vi "Main.vi"(7 "sweep rate, /min":dbl=0.2, 8 "sweep to:":dbl=-0.5, 9 "sweep":T3(radio)=enum."time_sweep") -> ()   [LabVIEW 2017] (continued)
                      n1646 = Number To Decimal String(number=w2143) -> (decimal integer string=w2142:string)  [unwired: 1 in]
                      n1647 = GPIB Write(0:w2142, 1:":SENSe:DATA:FRES?") -> (6:w2147:errorcluster)  [unwired: 3 in, 1 out]
                      n1648 = GPIB Read(0:w2142, 1:200, 3:w2147) -> (5:w2141:string)  [unwired: 2 in, 2 out]
                      n1649 = Fract/Exp String To Number(string=w2141) -> (number=w2145:dbl)  [unwired: 3 in, 1 out]
                      n1650 = Build Array (concatenate)(w2149, w2145) -> (w2148:dbl[])
                    }
                  }
                  n1651 = property on="data" class="Arr (strict)"("Value"=w2139) -> ()  [unwired: 2 in, 2 out]
                }
                frame #17 {
                  # "check if 2nd channel \non Keithley 2182A 2\nis to be measured"
                  n1652 = property on="data" class="Arr (strict)"() -> ("Value"=w2151:dbl[])  [unwired: 2 in, 2 out]
                  n1653 = local read "2182A 2 ch2"() -> (w2150:bool)
                  n1654 = case shown="True" w2150 {
                    tunnel: w2151 -> [w2153 w2166]
                    tunnel: [w2153 w2165] -> w2152
                    frame False {
                      # "we are not measuring 2182A 2 channel 2 (2182A_2_ch2)"
                    }
                    frame True {
                      # "switching to channel 2 and then\nback to channel 1"
                      # "we are  measuring 2182A 2 channel 2 (2182A_2_ch2)"
                      n1655 = local read "2182A 2 addr"() -> (w2160:u8)
                      n1656 = Number To Decimal String(number=w2160) -> (decimal integer string=w2155:string)  [unwired: 1 in]
                      n1657 = GPIB Write(0:w2155, 1:":SENSe:CHAN 2") -> (6:w2157:errorcluster)  [unwired: 3 in, 1 out]
                      n1658 = GPIB Write(0:w2155, 1:":SENSe:DATA:FRES?", 3:w2157) -> (6:w2164:errorcluster)  [unwired: 2 in, 1 out]
                      n1659 = GPIB Read(0:w2155, 1:200, 3:w2164) -> (5:w2159:string, 7:w2156:errorcluster)  [unwired: 2 in, 1 out]
                      n1660 = GPIB Write(0:w2155, 1:":SENSe:CHAN 1", 3:w2156) -> ()  [unwired: 2 in, 2 out]
                      n1661 = Fract/Exp String To Number(string=w2159) -> (number=w2162:dbl)  [unwired: 3 in, 1 out]
                      n1662 = Build Array (concatenate)(w2166, w2162) -> (w2165:dbl[])
                    }
                  }
                  n1663 = property on="data" class="Arr (strict)"("Value"=w2152) -> ()  [unwired: 2 in, 2 out]
                }
                frame #18 {
                  # "check if 1st channel \non Keithley 2182A 3\nis to be measured"
                  n1664 = property on="data" class="Arr (strict)"() -> ("Value"=w2168:dbl[])  [unwired: 2 in, 2 out]
                  n1665 = local read "2182A 3 ch1"() -> (w2167:bool)
                  n1666 = case shown="True" w2167 {
                    tunnel: w2168 -> [w2170 w2179]
                    tunnel: [w2170 w2178] -> w2169
                    frame False {
                      # "we are not measuring 2182A 3 channel 1 (2182A_3_ch1)"
                    }
                    frame True {
                      # "we are  measuring 2182A 3 channel 1 (2182A_3_ch1)"
                      n1667 = local read "2182A 3 addr"() -> (w2173:u8)
                      n1668 = Number To Decimal String(number=w2173) -> (decimal integer string=w2172:string)  [unwired: 1 in]
                      n1669 = GPIB Write(0:w2172, 1:":SENSe:DATA:FRES?") -> (6:w2177:errorcluster)  [unwired: 3 in, 1 out]
                      n1670 = GPIB Read(0:w2172, 1:200, 3:w2177) -> (5:w2171:string)  [unwired: 2 in, 2 out]
                      n1671 = Fract/Exp String To Number(string=w2171) -> (number=w2175:dbl)  [unwired: 3 in, 1 out]
                      n1672 = Build Array (concatenate)(w2179, w2175) -> (w2178:dbl[])
                    }
                  }
                  n1673 = property on="data" class="Arr (strict)"("Value"=w2169) -> ()  [unwired: 2 in, 2 out]
                }
                frame #19 {
                  # "check if 2nd channel \non Keithley 2182A 3\nis to be measured"
                  n1674 = property on="data" class="Arr (strict)"() -> ("Value"=w2181:dbl[])  [unwired: 2 in, 2 out]
                  n1675 = local read "2182A 3 ch2"() -> (w2180:bool)
                  n1676 = case shown="True" w2180 {
                    tunnel: w2181 -> [w2183 w2196]
                    tunnel: [w2183 w2195] -> w2182
                    frame False {
                      # "we are not measuring 2182A 3 channel 2 (2182A_3_ch2)"
                    }
                    frame True {
                      # "switching to channel 2 and then\nback to channel 1"
                      # "we are  measuring 2182A 3 channel 2 (2182A_3_ch2)"
                      n1677 = local read "2182A 3 addr"() -> (w2190:u8)
                      n1678 = Number To Decimal String(number=w2190) -> (decimal integer string=w2185:string)  [unwired: 1 in]
                      n1679 = GPIB Write(0:w2185, 1:":SENSe:CHAN 2") -> (6:w2187:errorcluster)  [unwired: 3 in, 1 out]
                      n1680 = GPIB Write(0:w2185, 1:":SENSe:DATA:FRES?", 3:w2187) -> (6:w2194:errorcluster)  [unwired: 2 in, 1 out]
                      n1681 = GPIB Read(0:w2185, 1:200, 3:w2194) -> (5:w2189:string, 7:w2186:errorcluster)  [unwired: 2 in, 1 out]
                      n1682 = GPIB Write(0:w2185, 1:":SENSe:CHAN 1", 3:w2186) -> ()  [unwired: 2 in, 2 out]
                      n1683 = Fract/Exp String To Number(string=w2189) -> (number=w2192:dbl)  [unwired: 3 in, 1 out]
                      n1684 = Build Array (concatenate)(w2196, w2192) -> (w2195:dbl[])
                    }
                  }
                  n1685 = property on="data" class="Arr (strict)"("Value"=w2182) -> ()  [unwired: 2 in, 2 out]
                }
                frame #20 {
                  # "check if 1st channel \non Keithley 2182A 4\nis to be measured"
                  n1686 = property on="data" class="Arr (strict)"() -> ("Value"=w2198:dbl[])  [unwired: 2 in, 2 out]
                  n1687 = local read "2182A 4 ch1"() -> (w2197:bool)
                  n1688 = case shown="True" w2197 {
                    tunnel: w2198 -> [w2200 w2209]
                    tunnel: [w2200 w2208] -> w2199
                    frame False {
                      # "we are not measuring 2182A 4 channel 1 (2182A_4_ch1)"
                    }
                    frame True {
                      # "we are  measuring 2182A 4 channel 1 (2182A_4_ch1)"
                      n1689 = local read "2182A 4 addr"() -> (w2203:u8)
                      n1690 = Number To Decimal String(number=w2203) -> (decimal integer string=w2202:string)  [unwired: 1 in]
                      n1691 = GPIB Write(0:w2202, 1:":SENSe:DATA:FRES?") -> (6:w2207:errorcluster)  [unwired: 3 in, 1 out]
                      n1692 = GPIB Read(0:w2202, 1:200, 3:w2207) -> (5:w2201:string)  [unwired: 2 in, 2 out]
                      n1693 = Fract/Exp String To Number(string=w2201) -> (number=w2205:dbl)  [unwired: 3 in, 1 out]
                      n1694 = Build Array (concatenate)(w2209, w2205) -> (w2208:dbl[])
                    }
                  }
                  n1695 = property on="data" class="Arr (strict)"("Value"=w2199) -> ()  [unwired: 2 in, 2 out]
                }
                frame #21 {
                  # "check if 2nd channel \non Keithley 2182A 4\nis to be measured"
                  n1696 = property on="data" class="Arr (strict)"() -> ("Value"=w2211:dbl[])  [unwired: 2 in, 2 out]
                  n1697 = local read "2182A 4 ch2"() -> (w2210:bool)
                  n1698 = case shown="True" w2210 {
                    tunnel: w2211 -> [w2213 w2226]
                    tunnel: [w2213 w2225] -> w2212
                    frame False {
                      # "we are not measuring 2182A 4 channel 2 (2182A_4_ch2)"
                    }
                    frame True {
                      # "switching to channel 2 and then\nback to channel 1"
                      # "we are  measuring 2182A 4 channel 2 (2182A_4_ch2)"
                      n1699 = local read "2182A 4 addr"() -> (w2220:u8)
                      n1700 = Number To Decimal String(number=w2220) -> (decimal integer string=w2215:string)  [unwired: 1 in]
                      n1701 = GPIB Write(0:w2215, 1:":SENSe:CHAN 2") -> (6:w2217:errorcluster)  [unwired: 3 in, 1 out]
                      n1702 = GPIB Write(0:w2215, 1:":SENSe:DATA:FRES?", 3:w2217) -> (6:w2224:errorcluster)  [unwired: 2 in, 1 out]
                      n1703 = GPIB Read(0:w2215, 1:200, 3:w2224) -> (5:w2219:string, 7:w2216:errorcluster)  [unwired: 2 in, 1 out]
                      n1704 = GPIB Write(0:w2215, 1:":SENSe:CHAN 1", 3:w2216) -> ()  [unwired: 2 in, 2 out]
                      n1705 = Fract/Exp String To Number(string=w2219) -> (number=w2222:dbl)  [unwired: 3 in, 1 out]
                      n1706 = Build Array (concatenate)(w2226, w2222) -> (w2225:dbl[])
                    }
                  }
                  n1707 = property on="data" class="Arr (strict)"("Value"=w2212) -> ()  [unwired: 2 in, 2 out]
                }
                frame #22 {
                  # "check if voltage on\nKeithley 2636A smua\nis to be measured"
                  n1708 = local read "2636A smua meas v"() -> (w2227:bool)
                  n1709 = property on="data" class="Arr (strict)"() -> ("Value"=w2228:dbl[])  [unwired: 2 in, 2 out]
                  n1710 = case shown="True" w2227 {
                    tunnel: w2228 -> [w2230 w2236]
                    tunnel: [w2230 w2235] -> w2229
                    frame False {
                      # "we are not measuring voltage on 2636A smua (2636A_smua_v)"
                    }
                    frame True {
                      # "we are  measuring voltage on 2636A smua (2636A_smua_v)"
                      n1711 = local read "2336A addr"() -> (w2231:refnum<visa-resource-name>)
                      n1712 = call "SinglePointMeasurement.vi"("Measure"=Measure."Voltage", "Channel"=Channel."a", "VISA resource name 2"=w2231) -> ("Measuremet"=w2233:dbl)  [unwired: 3 in, 4 out]
                      n1713 = Build Array (concatenate)(w2236, w2233) -> (w2235:dbl[])
                    }
                  }
                  n1714 = property on="data" class="Arr (strict)"("Value"=w2229) -> ()  [unwired: 2 in, 2 out]
                }
                frame #23 {
                  # "check if current on\nKeithley 2636A smua\nis to be measured"
                  n1715 = local read "2636A smua meas i"() -> (w2237:bool)
                  n1716 = property on="data" class="Arr (strict)"() -> ("Value"=w2238:dbl[])  [unwired: 2 in, 2 out]
                  n1717 = case shown="True" w2237 {
                    tunnel: w2238 -> [w2240 w2243]
                    tunnel: [w2240 w2242] -> w2239
                    frame False {
                      # "we are not measuring current on 2636A smua (2636A_smua_i)"
                    }
                    frame True {
                      # "we are  measuring current on 2636A smua (2636A_smua_i)"
                      n1718 = stacked-sequence {
                        tunnel: [_ w2252] -> w2241
                        frame #0 {
                          n1719 = local read "auto\nrange A"() -> (w2247:bool)
                          n1720 = local read "2336A addr"() -> (w2250:refnum<visa-resource-name>)
                          n1721 = Select(t="smua.AUTORANGE_ON", s=w2247, f="smua.AUTORANGE_OFF") -> (s? t:f=w2245:string)
                          n1722 = Concatenate Strings("smua.measure.autorangei = ", w2245) -> (w2244:string)
                          n1723 = VISA Write(VISA resource name=w2250, write buffer=w2244) -> ()  [unwired: 1 in, 3 out]
                        }
                        frame #1 {
                          n1724 = local read "2336A addr"() -> (w2254:refnum<visa-resource-name>)
                          n1725 = call "SinglePointMeasurement.vi"("Measure"=Measure."Current", "Channel"=Channel."a", "VISA resource name 2"=w2254) -> ("Measuremet"=w2252:dbl)  [unwired: 3 in, 4 out]
                        }
                      }
                      n1726 = Build Array (concatenate)(w2243, w2241) -> (w2242:dbl[])
                    }
                  }
                  n1727 = property on="data" class="Arr (strict)"("Value"=w2239) -> ()  [unwired: 2 in, 2 out]
                }
                frame #24 {
                  # "check if voltage on\nKeithley 2636A smub\nis to be measured"
                  n1728 = local read "2636A smub meas v"() -> (w2255:bool)
                  n1729 = property on="data" class="Arr (strict)"() -> ("Value"=w2256:dbl[])  [unwired: 2 in, 2 out]
                  n1730 = case shown="True" w2255 {
                    tunnel: w2256 -> [w2258 w2264]
                    tunnel: [w2258 w2263] -> w2257
                    frame False {
                      # "we are not measuring voltage on 2636A smub (2636A_smub_v)"
                    }
                    frame True {
                      # "we are  measuring voltage on 2636A smub (2636A_smub_v)"
                      n1731 = local read "2336A addr"() -> (w2262:refnum<visa-resource-name>)
                      n1732 = call "SinglePointMeasurement.vi"("Measure"=Measure."Voltage", "Channel"=Channel."b", "VISA resource name 2"=w2262) -> ("Measuremet"=w2260:dbl)  [unwired: 3 in, 4 out]
                      n1733 = Build Array (concatenate)(w2264, w2260) -> (w2263:dbl[])
                    }
                  }
                  n1734 = property on="data" class="Arr (strict)"("Value"=w2257) -> ()  [unwired: 2 in, 2 out]
                }
                frame #25 {
                  # "check if current on\nKeithley 2636A smub\nis to be measured"
                  n1735 = local read "2636A smub meas i"() -> (w2265:bool)
                  n1736 = property on="data" class="Arr (strict)"() -> ("Value"=w2266:dbl[])  [unwired: 2 in, 2 out]
                  n1737 = case shown="True" w2265 {
                    tunnel: w2266 -> [w2268 w2271]
                    tunnel: [w2268 w2270] -> w2267
                    frame False {
                      # "we are not measuring current on 2636A smub (2636A_smub_i)"
                    }
                    frame True {
                      # "we are  measuring current on 2636A smub (2636A_smub_i)"
                      n1738 = stacked-sequence {
                        tunnel: [_ w2280] -> w2269
                        frame #0 {
                          n1739 = local read "auto\nrange B"() -> (w2275:bool)
                          n1740 = local read "2336A addr"() -> (w2278:refnum<visa-resource-name>)
                          n1741 = Select(t="smub.AUTORANGE_ON", s=w2275, f="smub.AUTORANGE_OFF") -> (s? t:f=w2273:string)
                          n1742 = Concatenate Strings("smub.measure.autorangei = ", w2273) -> (w2272:string)
                          n1743 = VISA Write(VISA resource name=w2278, write buffer=w2272) -> ()  [unwired: 1 in, 3 out]
                        }
                        frame #1 {
                          n1744 = local read "2336A addr"() -> (w2282:refnum<visa-resource-name>)
                          n1745 = call "SinglePointMeasurement.vi"("Measure"=Measure."Current", "Channel"=Channel."b", "VISA resource name 2"=w2282) -> ("Measuremet"=w2280:dbl)  [unwired: 3 in, 4 out]
                        }
                      }
                      n1746 = Build Array (concatenate)(w2271, w2269) -> (w2270:dbl[])
                    }
                  }
                  n1747 = property on="data" class="Arr (strict)"("Value"=w2267) -> ()  [unwired: 2 in, 2 out]
                }
                frame #26 {
                  # "check if time\nis to be measured"
                  n1748 = property on="data" class="Arr (strict)"() -> ("Value"=w2285:dbl[])  [unwired: 2 in, 2 out]
                  n1749 = local read "measure time"() -> (w2284:bool)
                  n1750 = case shown="True" w2284 {
                    tunnel: w2285 -> [w2287 w2293]
                    tunnel: [w2287 w2292] -> w2286
                    tunnel: w2283 -> [_ w2290]
                    frame False {
                      # "we are not measuring time"
                    }
                    frame True {
                      # "seconds from the beginning of month"
                      # "we are  measuring time"
                      n1751 = call "timeInSeconds.vi"() -> ("Numeric"=w2291:dbl, "current time"=w2288:timestamp)  [unwired: 2 in]
                      n1752 = property on="current time" class="AbsTime (strict)"("Value"=w2288) -> ()  [unwired: 2 in, 2 out]
                      n1753 = Subtract(x=w2291, y=w2290) -> (x-y=w2289:dbl)
                      n1754 = Build Array (concatenate)(w2293, w2289) -> (w2292:dbl[])
                    }
                  }
                  n1755 = property on="data" class="Arr (strict)"("Value"=w2286) -> ()  [unwired: 2 in, 2 out]
                }
                frame #27 {
                  n1756 = local read "iPS_MagnetField"() -> (w2294:bool)
                  n1757 = property on="data" class="Arr (strict)"() -> ("Value"=w2295:dbl[])  [unwired: 2 in, 2 out]
                  n1758 = case shown="True" w2294 {
                    tunnel: w2295 -> [w2297 w2306]
                    tunnel: [w2297 w2305] -> w2296
                    frame False {
                      # "we are not Measuring magnetic field on IPS120-0"
                    }
                    frame True {
                      w2301 = 1
                      # "Measure magnetic field on Teslatron_iPS_Field"
                      n1759 = local read "IPS120-0 addr_sweep"() -> (w2304:u8)
                      n1760 = Number To Decimal String(number=w2304) -> (decimal integer string=w2303:string)  [unwired: 1 in]
                      n1761 = GPIB Write(0:w2303, 1:"R 7", 2:w2301) -> ()  [unwired: 2 in, 2 out]
                      n1762 = GPIB Read(0:w2303, 1:200 ("byte count"), 2:w2301) -> (5:w2299:string)  [unwired: 2 in, 2 out]
                      n1763 = Fract/Exp String To Number(string=w2299, offset=w2301) -> (number=w2300:dbl)  [unwired: 2 in, 1 out]
                      n1764 = Build Array (concatenate)(w2306, w2300) -> (w2305:dbl[])
                    }
                  }
                  n1765 = property on="data" class="Arr (strict)"("Value"=w2296) -> ()  [unwired: 2 in, 2 out]
                }
                frame #28 {
                  # "check if current \non 2461 SouceMeter\nis to be measured"
                  n1766 = property on="data" class="Arr (strict)"() -> ("Value"=w2308:dbl[])  [unwired: 2 in, 2 out]
                  n1767 = property on="iTC_Sample_T" class="Bool (strict)"() -> ("Value"=w2307:bool)  [unwired: 2 in, 2 out]
                  n1768 = case shown="True" w2307 {
                    tunnel: w2308 -> [w2310 w2323]
                    tunnel: [w2310 w2322] -> w2309
                    frame False {
                      # "we are not measuring 2461, voltage (2461_meas_v)"
                    }
                    frame True {
                      w2316 = 1
                      # "temporarily ITC503S"
                      # "we are  measuring Sample_T"
                      n1769 = property on="iTC_503_addr_sweep" class="DigNum (strict)"() -> ("Value"=w2311:u8)  [unwired: 2 in, 2 out]
                      n1770 = Number To Decimal String(number=w2311) -> (decimal integer string=w2312:string)  [unwired: 1 in]
                      n1771 = GPIB Write(0:w2312, 1:"$C3", 2:1) -> (6:w2319:errorcluster)  [unwired: 2 in, 1 out]
                      n1772 = GPIB Write(0:w2312, 1:"R3", 2:w2316, 3:w2319) -> (6:w2321:errorcluster)  [unwired: 1 in, 1 out]
                      n1773 = GPIB Read(0:w2312, 1:200, 2:w2316, 3:w2321) -> (5:w2320:string)  [unwired: 1 in, 2 out]
                      n1774 = Fract/Exp String To Number(string=w2320, offset=w2316) -> (number=w2313:dbl)  [unwired: 2 in, 1 out]
                      n1775 = Build Array (concatenate)(w2323, w2313) -> (w2322:dbl[])
                    }
                  }
                  n1776 = property on="data" class="Arr (strict)"("Value"=w2309) -> ()  [unwired: 2 in, 2 out]
                }
                frame #29 {
                  # "check if current \non 2461 SouceMeter\nis to be measured"
                  n1777 = property on="CH_A" class="Bool (strict)"() -> ("Value"=w2324:bool)  [unwired: 2 in, 2 out]
                  n1778 = property on="data" class="Arr (strict)"() -> ("Value"=w2325:dbl[])  [unwired: 2 in, 2 out]
                  n1779 = case shown="True" w2324 {
                    tunnel: w2325 -> [w2327 w2340]
                    tunnel: [w2327 w2339] -> w2326
                    frame False {
                      # "we are not measuring 2461, voltage (2461_meas_v)"
                    }
                    frame True {
                      w2333 = 1
                      # "temporarily ITC503S"
                      # "we are  measuring iTC503_CHA"
                      n1780 = property on="iTC_503_addr_sweep" class="DigNum (strict)"() -> ("Value"=w2328:u8)  [unwired: 2 in, 2 out]
                      n1781 = Number To Decimal String(number=w2328) -> (decimal integer string=w2329:string)  [unwired: 1 in]
                      n1782 = GPIB Write(0:w2329, 1:"$C3", 2:1) -> (6:w2336:errorcluster)  [unwired: 2 in, 1 out]
                      n1783 = GPIB Write(0:w2329, 1:"R3", 2:w2333, 3:w2336) -> (6:w2338:errorcluster)  [unwired: 1 in, 1 out]
                      n1784 = GPIB Read(0:w2329, 1:200, 2:w2333, 3:w2338) -> (5:w2337:string)  [unwired: 1 in, 2 out]
                      n1785 = Fract/Exp String To Number(string=w2337, offset=w2333) -> (number=w2330:dbl)  [unwired: 2 in, 1 out]
                      n1786 = Build Array (concatenate)(w2340, w2330) -> (w2339:dbl[])
                    }
                  }
                  n1787 = property on="data" class="Arr (strict)"("Value"=w2326) -> ()  [unwired: 2 in, 2 out]
                }
                frame #30 {
                  # "check if current \non 2461 SouceMeter\nis to be measured"
                  n1788 = property on="CH_B" class="Bool (strict)"() -> ("Value"=w2341:bool)  [unwired: 2 in, 2 out]
                  n1789 = property on="data" class="Arr (strict)"() -> ("Value"=w2342:dbl[])  [unwired: 2 in, 2 out]
                  n1790 = case shown="True" w2341 {
                    tunnel: w2342 -> [w2344 w2357]
                    tunnel: [w2344 w2356] -> w2343
                    frame False {
                      # "we are not measuring 2461, voltage (2461_meas_v)"
                    }
                    frame True {
                      w2350 = 1
                      # "temporarily ITC503S"
                      # "we are  measuring iTC503_CHA"
                      n1791 = property on="iTC_503_addr_sweep" class="DigNum (strict)"() -> ("Value"=w2345:u8)  [unwired: 2 in, 2 out]
                      n1792 = Number To Decimal String(number=w2345) -> (decimal integer string=w2346:string)  [unwired: 1 in]
                      n1793 = GPIB Write(0:w2346, 1:"$C3", 2:1) -> (6:w2353:errorcluster)  [unwired: 2 in, 1 out]
                      n1794 = GPIB Write(0:w2346, 1:"R2", 2:w2350, 3:w2353) -> (6:w2355:errorcluster)  [unwired: 1 in, 1 out]
                      n1795 = GPIB Read(0:w2346, 1:200, 2:w2350, 3:w2355) -> (5:w2354:string)  [unwired: 1 in, 2 out]
                      n1796 = Fract/Exp String To Number(string=w2354, offset=w2350) -> (number=w2347:dbl)  [unwired: 2 in, 1 out]
                      n1797 = Build Array (concatenate)(w2357, w2347) -> (w2356:dbl[])
                    }
                  }
                  n1798 = property on="data" class="Arr (strict)"("Value"=w2343) -> ()  [unwired: 2 in, 2 out]
                }
                frame #31 {
                  # "Record Step Value \nif it is mapping"
                  n1799 = property on="Linetrace or Mapping?" class="Bool (strict)"() -> ("Value"=w2359:bool)  [unwired: 2 in, 2 out]
                  n1800 = property on="data" class="Arr (strict)"() -> ("Value"=w2360:dbl[])  [unwired: 2 in, 2 out]
                  n1801 = case shown="True" w2359 {
                    tunnel: w2360 -> [w2361 w2364]
                    tunnel: [w2361 w2363] -> w2358
                    frame False {
                      # "We are not recording Step Value if it is linetrace"
                    }
                    frame True {
                      # "We are recording Step Value if it is mapping"
                      n1802 = property on="Current Step Value" class="DigNum (strict)"() -> ("Value"=w2362:dbl)  [unwired: 2 in, 2 out]
                      n1803 = Build Array (concatenate)(w2364, w2362) -> (w2363:dbl[])
                    }
                  }
                  n1804 = property on="data" class="Arr (strict)"("Value"=w2358) -> ()  [unwired: 2 in, 2 out]
                }
              }
            }
            frame #4 {
              # "this part appends last\nmeasured point to the \ndata file"
              n1805 = local read "Data file:"() -> (w2366:path)
              n1806 = property on="data" class="Arr (strict)"() -> ("Value"=w2365:dbl[])  [unwired: 2 in, 2 out]
              n1807 = call-poly <vilib>:"Write To Spreadsheet File.vi"("format (%.3f)"="%.6e", "append to file? (new file:F)"=TRUE, "1D data"=w2365, "file path (dialog if empty)"=w2366) -> ()  [unwired: 4 in, 1 out]
            }
            frame #5 {
              n1808 = property on="data" class="Arr (strict)"() -> ("Value"=w2369:dbl[])  [unwired: 2 in, 2 out]
            }
          }
          n1809 = stacked-sequence "add data to array" {
            tunnel: w1878 -> [w2498]
            tunnel: [w2497] -> w1877
            tunnel: w1863 -> [w2496]
            frame #0 {
              n1810 = Build Array (concatenate)(w2498, w2496) -> (w2497:dbl[][])
            }
          }
          n1811 = And(x=w1865, y="Continuous Sweep") -> (x .and. y?=w1870:bool)
          n1812 = case shown="True" w1870 {
            frame False {
            }
            frame True {
              n1813 = property on="upper limit" class="DigNum (strict)"() -> ("Value"=w1879:dbl)  [unwired: 2 in, 2 out]
              n1814 = local read "sweep to:"() -> (w1881:dbl)
              n1815 = property on="lower limit" class="DigNum (strict)"() -> ("Value"=w1880:dbl)  [unwired: 2 in, 2 out]
              n1816 = Equal?(x=w1881, y=w1879) -> (x = y?=w1882:bool)
              n1817 = Select(t=w1880, s=w1882, f=w1879) -> (s? t:f=w1883:dbl)
              n1818 = local write "sweep to:"(w1883) -> ()
            }
          }
          n1819 = stacked-sequence "plot selected measurements" {
            seq-local: [_ w2521 _] -> [_ _ w2566]
            seq-local: [_ w2520 _] -> [_ _ w2567]
            tunnel: w1877 -> [_ w2519 _]
            frame #0 {
              n1820 = property on="XY Graph" class="XYGraph (strict)"("ActYScl"=0 ("Active Y Scale")) -> (error out=w2504:errorcluster)  [unwired: 2 in, 1 out]
              n1821 = property on="Show cursor" class="Bool (strict)"() -> ("Value"=w2499:bool)  [unwired: 2 in, 2 out]
              n1822 = property on="Xaxis" class="Ring (strict)"() -> ("Value"=w2509:u16)  [unwired: 2 in, 2 out]
              n1823 = property on="Yaxis" class="Ring (strict)"(error in=w2504) -> (error out=w2503:errorcluster, "RingText.Text"=w2502:string)  [unwired: 1 in, 1 out]
              n1824 = property on="XY Graph" class="XYGraph (strict)"("Cursor.Visible"=w2499) -> ()  [unwired: 2 in, 2 out]
              n1825 = property on="Figure_axis" class="Arr (strict)"() -> ("Value"=w2510:string[])  [unwired: 2 in, 2 out]
              n1826 = property on="XY Graph" class="XYGraph (strict)"(error in=w2503, "YScale.NameLbl.Text"=w2502) -> (error out=w2500:errorcluster)  [unwired: 1 in, 1 out]
              n1827 = property on="XY Graph" class="XYGraph (strict)"(error in=w2500, "ActYScl"=1 ("Active Y Scale")) -> (error out=w2506:errorcluster)  [unwired: 1 in, 1 out]
              n1828 = property on="Yright" class="Ring (strict)"(error in=w2506) -> (error out=w2507:errorcluster, "RingText.Text"=w2501:string)  [unwired: 1 in, 1 out]
              n1829 = Index Array(array=w2510, index=w2509) -> (element=w2511:string)
              n1830 = property on="XY Graph" class="XYGraph (strict)"("XScale.NameLbl.Text"=w2511) -> ()  [unwired: 2 in, 2 out]
              n1831 = property on="XY Graph" class="XYGraph (strict)"(error in=w2507, "YScale.NameLbl.Text"=w2501) -> ()  [unwired: 1 in, 2 out]
            }
            frame #1 {
              n1832 = local read "Xaxis"() -> (w2524:u16)
              n1833 = property on="Yright" class="Ring (strict)"() -> ("Value"=w2518:u16)  [unwired: 2 in, 2 out]
              n1834 = property on="Yright" class="Ring (strict)"() -> ("RingText.Text"=w2517:string)  [unwired: 2 in, 2 out]
              n1835 = property on="Xaxis" class="Ring (strict)"() -> ("RingText.Text"=w2523:string)  [unwired: 2 in, 2 out]
              n1836 = property on="Yaxis" class="Ring (strict)"() -> ("RingText.Text"=w2522:string)  [unwired: 2 in, 2 out]
              n1837 = local read "Yaxis"() -> (w2525:u16)
              n1838 = case shown="\"formula\"" w2517 {
                tunnel: [w2530 w2537] -> w2515
                tunnel: w2518 -> [_ w2536]
                tunnel: w2519 -> [w2531 w2535]
                tunnel: [w2529 errorcluster {"status"=FALSE, "code"=0, "source"=""} ("error out")] -> _
                frame "formula" {
                  n1839 = local read "formula_variables"() -> (w2532:string[])
                  n1840 = Transpose 2D Array(2D array=w2531) -> (transposed array=w2533:dbl[][])
                  n1841 = property on="Y_right_formula" class="Str"() -> ("Value"=w2528:string)  [unwired: 2 in, 2 out]
                  n1842 = call <vilib>:"Eval Multi-Variable Array.vi"("Variables"=w2532, "X Values"=w2533, "formula"=w2528) -> ("error out"=w2529:errorcluster, "Y Values"=w2530:dbl[])  [unwired: 1 in]
                }
                frame "0", Default {
                  n1843 = Index Array(array=w2535, index (col)=w2536) -> (element=w2537:dbl[])  [unwired: 1 in]
                }
              }
              n1844 = case shown="\"formula\"" w2523 {
                tunnel: [w2548 w2553] -> w2527
                tunnel: w2524 -> [w2551 _]
                tunnel: w2519 -> [w2550 w2557]
                tunnel: [errorcluster {"status"=FALSE, "code"=0, "source"=""} ("error out") w2554] -> w2521
                tunnel: [w2548 w2553] -> w2516
                frame "0", Default {
                  n1845 = Index Array(array=w2550, index (col)=w2551) -> (element=w2548:dbl[])  [unwired: 1 in]
                }
                frame "formula" {
                  n1846 = local read "formula_variables"() -> (w2556:string[])
                  n1847 = Transpose 2D Array(2D array=w2557) -> (transposed array=w2555:dbl[][])
                  n1848 = property on="X_axis_formula" class="Str"() -> ("Value"=w2552:string)  [unwired: 2 in, 2 out]
                  n1849 = call <vilib>:"Eval Multi-Variable Array.vi"("Variables"=w2556, "X Values"=w2555, "formula"=w2552) -> ("error out"=w2554:errorcluster, "Y Values"=w2553:dbl[])  [unwired: 1 in]
                }
              }
              n1850 = case shown="\"formula\"" w2522 {
                tunnel: [w2540 w2547] -> w2526
                tunnel: w2525 -> [_ w2546]
                tunnel: w2519 -> [w2541 w2545]
                tunnel: [w2539 errorcluster {"status"=FALSE, "code"=0, "source"=""} ("error out")] -> w2520
                frame "formula" {
                  n1851 = local read "formula_variables"() -> (w2542:string[])
                  n1852 = Transpose 2D Array(2D array=w2541) -> (transposed array=w2543:dbl[][])
                  n1853 = property on="Y_left_formula" class="Str"() -> ("Value"=w2538:string)  [unwired: 2 in, 2 out]
                  n1854 = call <vilib>:"Eval Multi-Variable Array.vi"("Variables"=w2542, "X Values"=w2543, "formula"=w2538) -> ("error out"=w2539:errorcluster, "Y Values"=w2540:dbl[])  [unwired: 1 in]
                }
                frame "0", Default {
                  n1855 = Index Array(array=w2545, index (col)=w2546) -> (element=w2547:dbl[])  [unwired: 1 in]
                }
              }
              n1856 = Bundle("Y Values"=w2527, "Y Values"=w2526) -> (w2514:cluster{"Y Values":dbl[], "Y Values":dbl[]})  [unwired: 1 in]
              n1857 = Bundle("Y Values"=w2516, "Y Values"=w2515) -> (w2513:cluster{"Y Values":dbl[], "Y Values":dbl[]})  [unwired: 1 in]
              n1858 = Build Array(w2514, w2513) -> (w2512:cluster{"Y Values":dbl[], "Y Values":dbl[]}[])
              n1859 = property on="XY Graph" class="XYGraph (strict)"("Value"=w2512) -> ()  [unwired: 2 in, 2 out]
            }
            frame #2 {
              # "show if formula \nis wrong"
              n1860 = property on="Yaxis" class="Ring (strict)"() -> ("RingText.Text"=w2563:string)  [unwired: 2 in, 2 out]
              n1861 = property on="XY Graph" class="XYGraph (strict)"("Active Plot"=u32 0, "Plot.Plot Name"=w2563) -> (error out=w2564:errorcluster)  [unwired: 2 in, 1 out]
              n1862 = property on="Yright" class="Ring (strict)"() -> ("RingText.Text"=w2561:string)  [unwired: 2 in, 2 out]
              n1863 = property on="XY Graph" class="XYGraph (strict)"(error in=w2564, "Active Plot"=u32 1, "Plot.Plot Name"=w2561) -> ()  [unwired: 1 in, 2 out]
              n1864 = Unbundle By Name(w2567) -> ("status"=w2560:bool)
              n1865 = Unbundle By Name(w2566) -> ("status"=w2559:bool)
              n1866 = Unbundle By Name(w2566) -> ("status"=w2558:bool)
              n1867 = property on="status 3" class="Bool (strict)"("Value"=w2558) -> ()  [unwired: 2 in, 2 out]
              n1868 = property on="status 2" class="Bool (strict)"("Value"=w2560) -> ()  [unwired: 2 in, 2 out]
              n1869 = property on="status" class="Bool (strict)"("Value"=w2559) -> ()  [unwired: 2 in, 2 out]
            }
          }
          n1870 = stacked-sequence "set next value in the sweep" {
            tunnel: w1876 -> [w2370 _]
            tunnel: [w2370 _] -> w1875
            tunnel: w1873 -> [_ w2491]
            tunnel: w1868 -> [w2374 _]
            frame #0 {
              n1871 = local read "sweep"() -> (w2377:T3)
              n1872 = property on="Sweep Channel" class="DigNum (strict)"("Value"=w2370) -> ()  [unwired: 2 in, 2 out]
              n1873 = property on="sweep value" class="DigNum (strict)"("Value"=w2370) -> ()  [unwired: 2 in, 2 out]
              n1874 = case shown="\"iPS\"" w2377 {
                tunnel: w2370 -> [w2390 w2398 w2404 w2413 w2435 _ w2436 w2459]
                tunnel: w2374 -> [_ _ _ w2411 _ _ _ _]
                frame "2400_1" {
                  # "sweep voltage on 2400 1"
                  n1875 = local read "2400 1 addr"() -> (w2392:u8)
                  n1876 = Number To Fractional String(number=w2390) -> (F-format string=w2396:string)  [unwired: 3 in]
                  n1877 = Concatenate Strings(":INIT:IMM; :SOUR:VOLT:LEV:IMM:AMPL " ("data"), w2396) -> (w2394:string)
                  n1878 = Number To Decimal String(number=w2392) -> (decimal integer string=w2391:string)  [unwired: 1 in]
                  n1879 = GPIB Write(0:w2391, 1:w2394, 2:i16 1 ("mode (0)")) -> ()  [unwired: 2 in, 2 out]
                }
                frame "2400_2" {
                  # "sweep curr on 2400 2"
                  n1880 = Number To Fractional String(number=w2398) -> (F-format string=w2403:string)  [unwired: 3 in]
                  n1881 = local read "2400 2 addr"() -> (w2400:u8)
                  n1882 = Concatenate Strings(":INIT:IMM; :SOUR:CURR:LEV:IMM:AMPL " ("data"), w2403) -> (w2401:string)
                  n1883 = Number To Decimal String(number=w2400) -> (decimal integer string=w2399:string)  [unwired: 1 in]
                  n1884 = GPIB Write(0:w2399, 1:w2401, 2:i16 1 ("mode (0)")) -> ()  [unwired: 2 in, 2 out]
                }
                frame "2400_3" {
                  # "sweep voltage on 2400 3"
                  n1885 = local read "2400 3 addr"() -> (w2406:u8)
                  n1886 = Number To Fractional String(number=w2404) -> (F-format string=w2410:string)  [unwired: 3 in]
                  n1887 = Concatenate Strings(":INIT:IMM; :SOUR:VOLT:LEV:IMM:AMPL " ("data"), w2410) -> (w2408:string)
                  n1888 = Number To Decimal String(number=w2406) -> (decimal integer string=w2405:string)  [unwired: 1 in]
                  n1889 = GPIB Write(0:w2405, 1:w2408, 2:i16 1 ("mode (0)")) -> ()  [unwired: 2 in, 2 out]
                }
                frame "2636a_smua" {
                  n1890 = case shown="True" "sweep" {
                    tunnel: w2413 -> [w2418 w2431]
                    tunnel: w2411 -> [w2415 _]
                    frame True {
                      w2416 = 30.0 ("y")
                      n1891 = Subtract(x=w2418, y=w2415) -> (x-y=w2417:dbl)
                      n1892 = Divide(x=w2417, y=w2416) -> (x/y=w2414:dbl)
                      n1893 = for {
                        N: w2416 -> [_]
                        tunnel: w2415 -> [w2424]
                        tunnel: w2414 -> [w2422]
                        i -> [w2423]
                        n1894 = Multiply(x=w2422, y=w2423) -> (x*y=w2421:dbl)
                        n1895 = local read "2336A addr"() -> (w2426:refnum<visa-resource-name>)
                        n1896 = Add(x=w2421, y=w2424) -> (x+y=w2420:dbl)
                        n1897 = call "setLevel.vi"("VISA resource name 2"=w2426, "Source"=Source."Voltage", "Channel"=Channel."a", "SourceLevel"=w2420) -> ()  [unwired: 1 in, 3 out]
                        n1898 = Wait (ms)(milliseconds to wait=u32 12) -> ()  [unwired: 1 out]
                      }
                    }
                    frame False {
                      # "sweep voltage on 2636a smua"
                      n1899 = local read "2336A addr"() -> (w2429:refnum<visa-resource-name>)
                      n1900 = call "setLevel.vi"("VISA resource name 2"=w2429, "Source"=Source."Voltage", "Channel"=Channel."a", "SourceLevel"=w2431) -> ()  [unwired: 1 in, 3 out]
                    }
                  }
                }
                frame "2636a_smub" {
                  # "sweep voltage on 2636b smua"
                  n1901 = local read "2336A addr"() -> (w2432:refnum<visa-resource-name>)
                  n1902 = call "setLevel.vi"("VISA resource name 2"=w2432, "Source"=Source."Voltage", "Channel"=Channel."b", "SourceLevel"=w2435) -> ()  [unwired: 1 in, 3 out]
                }
                frame "time_sweep", Default {
                  # "do not sweep, just time"
                }
                frame "iPS" {
                  n1903 = stacked-sequence {
                    tunnel: w2436 -> [_ _ _ _ w2450 _ _]
                    frame #0 {
                      n1904 = local read "IPS120-0 addr_sweep"() -> (w2440:u8)
                      n1905 = Number To Decimal String(number=w2440) -> (decimal integer string=w2439:string)  [unwired: 1 in]
                      n1906 = GPIB Write(0:w2439, 1:"$C3", 2:i16 1 ("mode (0)")) -> ()  [unwired: 2 in, 2 out]
                    }
                    frame #1 {
                      n1907 = Wait (ms)(milliseconds to wait=u32 100) -> ()  [unwired: 1 out]
                    }
                    frame #2 {
                      n1908 = local read "IPS120-0 addr_sweep"() -> (w2445:u8)
                      n1909 = Number To Decimal String(number=w2445) -> (decimal integer string=w2444:string)  [unwired: 1 in]
                      n1910 = GPIB Write(0:w2444, 1:"$A1", 2:i16 1 ("mode (0)")) -> ()  [unwired: 2 in, 2 out]
                    }
                    frame #3 {
                      n1911 = Wait (ms)(milliseconds to wait=u32 100) -> ()  [unwired: 1 out]
                    }
                    frame #4 {
                      n1912 = Number To Fractional String(number=w2450) -> (F-format string=w2448:string)  [unwired: 3 in]
                      n1913 = local read "IPS120-0 addr_sweep"() -> (w2453:u8)
                      n1914 = Concatenate Strings("$J", w2448) -> (w2449:string)
                      n1915 = Number To Decimal String(number=w2453) -> (decimal integer string=w2452:string)  [unwired: 1 in]
                      n1916 = GPIB Write(0:w2452, 1:w2449, 2:i16 1 ("mode (0)")) -> ()  [unwired: 2 in, 2 out]
                    }
                    frame #5 {
                      n1917 = Wait (ms)(milliseconds to wait=u32 100) -> ()  [unwired: 1 out]
                    }
                    frame #6 {
                      n1918 = local read "IPS120-0 addr_sweep"() -> (w2458:u8)
                      n1919 = Number To Decimal String(number=w2458) -> (decimal integer string=w2457:string)  [unwired: 1 in]
                      n1920 = GPIB Write(0:w2457, 1:"$C2", 2:i16 1 ("mode (0)")) -> ()  [unwired: 2 in, 2 out]
                    }
                  }
                }
                frame "iTC" {
                  n1921 = stacked-sequence {
                    tunnel: w2459 -> [w2469 w2472]
                    frame #0 {
                      n1922 = property on="iTC_503_addr_sweep" class="DigNum (strict)"() -> ("Value"=w2460:u8)  [unwired: 2 in, 2 out]
                      n1923 = Less Or Equal To 0?(x=w2469) -> (x <= 0?=w2471:bool)
                      n1924 = Select(t=0.0, s=w2471, f=w2469) -> (s? t:f=w2461:dbl)
                      n1925 = Number To Decimal String(number=w2460) -> (decimal integer string=w2466:string)  [unwired: 1 in]
                      n1926 = Number To Fractional String(number=w2461, width (-)=5, precision (6)=4) -> (F-format string=w2468:string)  [unwired: 1 in]
                      n1927 = Concatenate Strings("$T ", w2468) -> (w2467:string)
                      n1928 = GPIB Write(0:w2466, 1:w2467, 2:3) -> ()  [unwired: 2 in, 2 out]
                    }
                    frame #1 {
                      n1929 = while {
                        tunnel: w2472 -> [w2485]
                        stop <- w2486 stop-if-true
                        w2477 = 1
                        n1930 = property on="iTC_503_addr_sweep" class="DigNum (strict)"() -> ("Value"=w2473:u8)  [unwired: 2 in, 2 out]
                        n1931 = Number To Decimal String(number=w2473) -> (decimal integer string=w2483:string)  [unwired: 1 in]
                        n1932 = GPIB Write(0:w2483, 1:"$C3", 2:1) -> (6:w2482:errorcluster)  [unwired: 2 in, 1 out]
                        n1933 = GPIB Write(0:w2483, 1:"R3", 2:w2477, 3:w2482) -> (6:w2480:errorcluster)  [unwired: 1 in, 1 out]
                        n1934 = GPIB Read(0:w2483, 1:200, 2:w2477, 3:w2480) -> (5:w2481:string)  [unwired: 1 in, 2 out]
                        n1935 = property on="Tolerance_Sweep" class="DigNum (strict)"() -> ("Value"=w2484:dbl)  [unwired: 2 in, 2 out]
                        n1936 = Fract/Exp String To Number(string=w2481, offset=w2477) -> (number=w2474:dbl)  [unwired: 2 in, 1 out]
                        n1937 = Subtract(x=w2474, y=w2485) -> (x-y=w2488:dbl)
                        n1938 = Absolute Value(x=w2488) -> (abs(x)=w2487:dbl)
                        n1939 = Less?(x=w2487, y=w2484) -> (x < y?=w2486:bool)
                      }
                    }
                  }
                }
              }
              n1940 = property on="Slope" class="DigNum (strict)"() -> ("Value"=w2371:dbl)  [unwired: 2 in, 2 out]
              n1941 = property on="Offset" class="DigNum (strict)"() -> ("Value"=w2373:dbl)  [unwired: 2 in, 2 out]
              n1942 = Multiply(x=w2371, y=w2370) -> (x*y=w2375:dbl)
              n1943 = Add(x=w2373, y=w2375) -> (x+y=w2376:dbl)
              n1944 = property on="Double Sweep" class="Bool (strict)"() -> ("Value"=w2372:bool)  [unwired: 2 in, 2 out]
              n1945 = case shown="True" w2372 {
                tunnel: w2376 -> [_ w2378]
                frame False {
                }
                frame True {
                  n1946 = disable-structure shown="Enabled" {
                    disable-tunnel: w2378 -> [w2379 w2387]
                    frame Disabled {
                      # "sweep voltage on 2400 2"
                      n1947 = local read "2400 2 addr"() -> (w2380:u8)
                      n1948 = Number To Fractional String(number=w2379) -> (F-format string=w2381:string)  [unwired: 3 in]
                      n1949 = Concatenate Strings(":INIT:IMM; :SOUR:VOLT:LEV:IMM:AMPL " ("data"), w2381) -> (w2383:string)
                      n1950 = Number To Decimal String(number=w2380) -> (decimal integer string=w2384:string)  [unwired: 1 in]
                      n1951 = GPIB Write(0:w2384, 1:w2383, 2:i16 1 ("mode (0)")) -> ()  [unwired: 2 in, 2 out]
                    }
                    frame Enabled {
                      n1952 = property on="Slave Channel" class="Enum (strict)"() -> ("Value"=w2386:T1)  [unwired: 2 in, 2 out]
                      n1953 = local read "2336A addr"() -> (w2389:refnum<visa-resource-name>)
                      n1954 = call "setLevel.vi"("VISA resource name 2"=w2389, "Source"=Source."Voltage", "Channel"=w2386, "SourceLevel"=w2387) -> ()  [unwired: 1 in, 3 out]
                    }
                  }
                }
              }
            }
            frame #1 {
              # "calculate deliberate time delay for the next step"
              n1955 = Tick Count (ms)() -> (millisecond timer value=w2493:u32)
              n1956 = Subtract(x=w2493, y=w2491) -> (x-y=w2492:u32)
              n1957 = property on="time/point, sec" class="DigNum (strict)"() -> ("Value"=w2494:dbl)  [unwired: 2 in, 2 out]
              n1958 = Multiply(x=w2494, y=1000.0) -> (x*y=w2490:dbl)
              n1959 = Subtract(x=w2490, y=w2492) -> (x-y=w2489:dbl)
              n1960 = property on="time delay, ms" class="DigNum (strict)"("Value"=w2489) -> ()  [unwired: 2 in, 2 out]
            }
          }
          n1961 = Not(x="Continuous Sweep") -> (.not. x?=w1869:bool)
          n1962 = And(x=w1865, y=w1869) -> (x .and. y?=w1867:bool)
          n1963 = Or(x=w1867, y="Stop Sweep") -> (x .or. y?=w1864:bool)
        }
        n1964 = stacked-sequence {
          tunnel: w1211 -> [_ _ _]
          tunnel: w1210 -> [_ _ w1837]
          frame #0 {
            n1965 = property on="Linetrace or Mapping?" class="Bool (strict)"() -> ("Value"=w1828:bool)  [unwired: 2 in, 2 out]
            n1966 = case shown="False" w1828 {
              frame False {
                w1830 = T5."Enabled" ("Disabled")
                w1829 = T5."Enabled" ("Disabled")
                # "Return the buttons to Idle state"
                n1967 = property on="sweep" class="RadioBtnsControl (strict)"("DisabledEnum"=w1829) -> ()  [unwired: 2 in, 2 out]
                n1968 = property on="2182A 1 addr" class="DigNum (strict)"("DisabledEnum"=w1829) -> ()  [unwired: 2 in, 2 out]
                n1969 = property on="2182A 2 addr" class="DigNum (strict)"("DisabledEnum"=w1829) -> ()  [unwired: 2 in, 2 out]
                n1970 = property on="2182A 3 addr" class="DigNum (strict)"("DisabledEnum"=w1829) -> ()  [unwired: 2 in, 2 out]
                n1971 = property on="2182A 4 addr" class="DigNum (strict)"("DisabledEnum"=w1829) -> ()  [unwired: 2 in, 2 out]
                n1972 = property on="2400 1 addr" class="DigNum (strict)"("DisabledEnum"=w1829) -> ()  [unwired: 2 in, 2 out]
                n1973 = property on="2400 2 addr" class="DigNum (strict)"("DisabledEnum"=w1829) -> ()  [unwired: 2 in, 2 out]
                n1974 = property on="2400 3 addr" class="DigNum (strict)"("DisabledEnum"=w1829) -> ()  [unwired: 2 in, 2 out]
                n1975 = property on="2336A addr" class="VISAName"("DisabledEnum"=w1829) -> ()  [unwired: 2 in, 2 out]
                n1976 = property on="SR830 1 addr" class="DigNum (strict)"("DisabledEnum"=w1829) -> ()  [unwired: 2 in, 2 out]
                n1977 = property on="SR830 2 addr" class="DigNum (strict)"("DisabledEnum"=w1829) -> ()  [unwired: 2 in, 2 out]
                n1978 = property on="SR830 3 addr" class="DigNum (strict)"("DisabledEnum"=w1829) -> ()  [unwired: 2 in, 2 out]
                n1979 = property on="SR830 4 addr" class="DigNum (strict)"("DisabledEnum"=w1829) -> ()  [unwired: 2 in, 2 out]
                n1980 = property on="sweep to:" class="DigNum (strict)"("DisabledEnum"=w1830) -> ()  [unwired: 2 in, 2 out]
                n1981 = property on="sweep rate, /min" class="DigNum (strict)"("DisabledEnum"=w1830) -> ()  [unwired: 2 in, 2 out]
              }
              frame True {
              }
            }
            n1982 = property on="Stop Sweep" class="Bool"("DisabledEnum"=T5."Disabled and Grayed Out" ("Disabled")) -> ()  [unwired: 2 in, 2 out]
          }
          frame #1 {
            n1983 = stacked-sequence {
              frame #0 {
                n1984 = local read "2636A smua meas v"() -> (w1835:bool)
                n1985 = local read "2636A smub meas v"() -> (w1833:bool)
                n1986 = local read "2636A smub meas i"() -> (w1832:bool)
                n1987 = local read "2636A smua meas i"() -> (w1834:bool)
                n1988 = Compound Arithmetic op=OR(w1835, w1834, w1833, w1832) -> (w1831:bool)
                n1989 = case shown="True" w1831 {
                  frame False {
                  }
                  frame True {
                    # "close session on 2636A"
                    n1990 = local read "2336A addr"() -> (w1836:refnum<visa-resource-name>)
                    n1991 = VISA Close(VISA resource name=w1836) -> ()  [unwired: 1 in, 1 out]
                  }
                }
              }
            }
          }
          frame #2 {
            n1992 = property on="Linetrace or Mapping?" class="Bool (strict)"() -> ("Value"=w1838:bool)  [unwired: 2 in, 2 out]
            n1993 = case shown="True" w1838 {
              tunnel: w1837 -> [w1841 w1844]
              frame False {
                w1839 = T5."Enabled" ("Disabled")
                n1994 = Enqueue Element(queue=w1841, element="Idle") -> ()  [unwired: 2 in, 3 out]
                n1995 = property on="Sweep Down" class="Bool"("DisabledEnum"=w1839) -> ()  [unwired: 2 in, 2 out]
                n1996 = property on="Sweep Up" class="Bool"("DisabledEnum"=w1839) -> ()  [unwired: 2 in, 2 out]
              }
              frame True {
                n1997 = property on="Sweep Direction" class="Str"() -> ("Value"=w1842:string)  [unwired: 2 in, 2 out]
                n1998 = case shown="\"Sweep Down\", Default" w1842 {
                  tunnel: w1844 -> [w1845 w1854]
                  frame "Sweep Down", Default {
                    n1999 = stacked-sequence {
                      tunnel: w1845 -> [_ _ w1852]
                      frame #0 {
                        n2000 = property on="Up Rate" class="DigNum (strict)"() -> ("Value"=w1848:dbl)  [unwired: 2 in, 2 out]
                        n2001 = property on="upper limit" class="DigNum (strict)"() -> ("Value"=w1847:dbl)  [unwired: 2 in, 2 out]
                        n2002 = property on="sweep to:" class="DigNum (strict)"("Value"=w1847) -> ()  [unwired: 2 in, 2 out]
                        n2003 = property on="sweep rate, /min" class="DigNum (strict)"("Value"=w1848) -> ()  [unwired: 2 in, 2 out]
                        n2004 = property on="Sweep Direction" class="Str"("Value"="Sweep Up" ("Sweep Direction")) -> ()  [unwired: 2 in, 2 out]
                      }
                      frame #1 {
                        n2005 = property on="wait between sweeps(s)" class="DigNum (strict)"() -> ("Value"=w1851:u32)  [unwired: 2 in, 2 out]
                        n2006 = Multiply(x=w1851, y=u32 1000) -> (x*y=w1850:u32)
                        n2007 = Wait (ms)(milliseconds to wait=w1850) -> ()  [unwired: 1 out]
                      }
                      frame #2 {
                        n2008 = Enqueue Element(queue=w1852, element="Step to Next Value") -> ()  [unwired: 2 in, 3 out]
                      }
                    }
                  }
                  frame "Sweep Up" {
                    n2009 = stacked-sequence {
                      tunnel: w1854 -> [_ w1862]
                      frame #0 {
                        n2010 = property on="Table Index" class="DigNum (strict)"() -> ("Value"=w1857:dbl)  [unwired: 2 in, 2 out]
                        n2011 = Increment(x=w1857) -> (x+1=w1856:dbl)
                        n2012 = property on="at field" class="Bool (strict)"("Value"=FALSE ("at field")) -> ()  [unwired: 2 in, 2 out]
                        n2013 = property on="Table Index" class="DigNum (strict)"("Value"=w1856) -> ()  [unwired: 2 in, 2 out]
                        n2014 = property on="lower limit" class="DigNum (strict)"() -> ("Value"=w1860:dbl)  [unwired: 2 in, 2 out]
                        n2015 = property on="Down Rate" class="DigNum (strict)"() -> ("Value"=w1859:dbl)  [unwired: 2 in, 2 out]
                        n2016 = property on="Sweep Direction" class="Str"("Value"="Sweep Down" ("Sweep Direction")) -> ()  [unwired: 2 in, 2 out]
                        n2017 = property on="sweep to:" class="DigNum (strict)"("Value"=w1860) -> ()  [unwired: 2 in, 2 out]
                        n2018 = property on="sweep rate, /min" class="DigNum (strict)"("Value"=w1859) -> ()  [unwired: 2 in, 2 out]
                      }
                      frame #1 {
                        n2019 = Enqueue Element(queue=w1862, element="Step to Next Value") -> ()  [unwired: 2 in, 3 out]
                      }
                    }
                  }
                }
                n2020 = property on="Sweep Down" class="Bool"("DisabledEnum"=T5."Disabled and Grayed Out" ("Disabled")) -> ()  [unwired: 2 in, 2 out]
              }
            }
          }
        }
      }
      frame "Ramp To Limit" {
        w2568 = dbl[][] []  # emty array for data
        # "0 = SR830_1_ip\n1 = SR830_1_oop\n2 = SR830_2_ip\n3 = SR830_2_oop\n4 = SR830_3_ip\n5 = SR830_3_oop\n6 = SR830_4_ip \n7 = SR830_4_oop \n8= 2400_1_v \n9 = 2400_1_i \n10 = 2400_2_v\n11 = 2400_2_i \n12 = 2400_3_v \n13 = 2400_3_i \n14 = 2182A_1_ch1 \n15 = 2182A_1_ch2 \n16 = 2182A_2_ch1 \n17 = 2182A_2_ch2\n18 = 2182A_3_ch1 \n19 = 2182A_3_ch2 \n20 = 2182A_4_ch1 \n21 = 2182A_4_ch2 \n22 = 2636A_smua_v \n23 = 2636A_smua_i \n24 = 2636A_smub_v \n25 = 2636A_smub_i \n26 = time\n27 = iPS_120\n28 = iTC _sample_T\n29 = iTC _CH_A\n30=iTC_CH_B\n31 = Step_Value"
        # "initial time in seconds\nfrom the beginning of month"
        n2021 = stacked-sequence {
          tunnel: [_ _ w3097 _ _] -> w2569
          frame #0 {
            n2022 = local read "2636A smua meas v"() -> (w2578:bool)
            n2023 = local read "2636A smub meas v"() -> (w2576:bool)
            n2024 = local read "2636A smub meas i"() -> (w2575:bool)
            n2025 = local read "2636A smua meas i"() -> (w2577:bool)
            n2026 = property on="sweep" class="RadioBtnsControl (strict)"() -> ("Value"=w2573:T3)  [unwired: 2 in, 2 out]
            n2027 = Compound Arithmetic op=OR(w2578, w2577, w2576, w2575) -> (w2574:bool)
            n2028 = case shown="\"time_sweep\", Default" w2573 {
              frame "2400_1" {
                # "add label for the first column in the datafile"
                n2029 = stacked-sequence {
                  frame #0 {
                    n2030 = property on="data_caption" class="Str"("Value"="") -> ()  [unwired: 2 in, 2 out]
                    n2031 = property on="Figure_axis" class="Arr (strict)"("Value"=string[] [] ("Figure_axis_string")) -> ()  [unwired: 2 in, 2 out]
                  }
                  frame #1 {
                    w2581 = "V_sweep_2400_1" ("V_sweep")
                    n2032 = Concatenate Strings(w2581, "\t") -> (w2583:string)
                    n2033 = Build Array(w2581) -> (w2582:string[])
                    n2034 = property on="data_caption" class="Str"("Value"=w2583) -> ()  [unwired: 2 in, 2 out]
                    n2035 = property on="Figure_axis" class="Arr (strict)"("Value"=w2582) -> ()  [unwired: 2 in, 2 out]
                  }
                }
              }
              frame "2400_2" {
                n2036 = stacked-sequence {
                  frame #0 {
                    n2037 = property on="data_caption" class="Str"("Value"="") -> ()  [unwired: 2 in, 2 out]
                    n2038 = property on="Figure_axis" class="Arr (strict)"("Value"=string[] [] ("Figure_axis_string")) -> ()  [unwired: 2 in, 2 out]
                  }
                  frame #1 {
                    w2587 = "V_sweep_2400_2" ("V_sweep")
                    n2039 = Build Array(w2587) -> (w2588:string[])
                    n2040 = Concatenate Strings(w2587, "\t") -> (w2590:string)
                    n2041 = property on="Figure_axis" class="Arr (strict)"("Value"=w2588) -> ()  [unwired: 2 in, 2 out]
                    n2042 = property on="data_caption" class="Str"("Value"=w2590) -> ()  [unwired: 2 in, 2 out]
                  }
                }
              }
              frame "2400_3" {
                n2043 = stacked-sequence {
                  frame #0 {
                    n2044 = property on="data_caption" class="Str"("Value"="") -> ()  [unwired: 2 in, 2 out]
                    n2045 = property on="Figure_axis" class="Arr (strict)"("Value"=string[] [] ("Figure_axis_string")) -> ()  [unwired: 2 in, 2 out]
                  }
                  frame #1 {
                    w2593 = "V_sweep_2400_3" ("V_sweep")
                    n2046 = Concatenate Strings(w2593, "\t") -> (w2596:string)
                    n2047 = Build Array(w2593) -> (w2594:string[])
                    n2048 = property on="data_caption" class="Str"("Value"=w2596) -> ()  [unwired: 2 in, 2 out]
                    n2049 = property on="Figure_axis" class="Arr (strict)"("Value"=w2594) -> ()  [unwired: 2 in, 2 out]
                  }
                }
              }
              frame "2636a_smua" {
                n2050 = stacked-sequence {
                  frame #0 {
                    n2051 = property on="data_caption" class="Str"("Value"="") -> ()  [unwired: 2 in, 2 out]
                    n2052 = property on="Figure_axis" class="Arr (strict)"("Value"=string[] [] ("Figure_axis_string")) -> ()  [unwired: 2 in, 2 out]
                  }
                  frame #1 {
                    w2599 = "V_sweep_2636a_smua" ("V_sweep")
                    n2053 = Concatenate Strings(w2599, "\t") -> (w2602:string)
                    n2054 = Build Array(w2599) -> (w2600:string[])
                    n2055 = property on="data_caption" class="Str"("Value"=w2602) -> ()  [unwired: 2 in, 2 out]
                    n2056 = property on="Figure_axis" class="Arr (strict)"("Value"=w2600) -> ()  [unwired: 2 in, 2 out]
                  }
                }
              }
              frame "2636a_smub" {
                n2057 = stacked-sequence {
                  frame #0 {
                    n2058 = property on="data_caption" class="Str"("Value"="") -> ()  [unwired: 2 in, 2 out]
                    n2059 = property on="Figure_axis" class="Arr (strict)"("Value"=string[] [] ("Figure_axis_string")) -> ()  [unwired: 2 in, 2 out]
                  }
                  frame #1 {
                    w2605 = "V_sweep_2636a_smub" ("V_sweep")
                    n2060 = Build Array(w2605) -> (w2606:string[])
                    n2061 = Concatenate Strings(w2605, "\t") -> (w2608:string)
                    n2062 = property on="Figure_axis" class="Arr (strict)"("Value"=w2606) -> ()  [unwired: 2 in, 2 out]
                    n2063 = property on="data_caption" class="Str"("Value"=w2608) -> ()  [unwired: 2 in, 2 out]
                  }
                }
              }
              frame "time_sweep", Default {
                n2064 = stacked-sequence {
                  frame #0 {
                    n2065 = property on="data_caption" class="Str"("Value"="") -> ()  [unwired: 2 in, 2 out]
                    n2066 = property on="Figure_axis" class="Arr (strict)"("Value"=string[] [] ("Figure_axis_string")) -> ()  [unwired: 2 in, 2 out]
                  }
                  frame #1 {
                    w2611 = "time_sweep" ("V_sweep")
                    n2067 = Build Array(w2611) -> (w2612:string[])
                    n2068 = Concatenate Strings(w2611, "\t") -> (w2613:string)
                    n2069 = property on="Figure_axis" class="Arr (strict)"("Value"=w2612) -> ()  [unwired: 2 in, 2 out]
                    n2070 = property on="data_caption" class="Str"("Value"=w2613) -> ()  [unwired: 2 in, 2 out]
                  }
                }
              }
              frame "iPS" {
                n2071 = stacked-sequence {
                  frame #0 {
                    n2072 = property on="data_caption" class="Str"("Value"="") -> ()  [unwired: 2 in, 2 out]
                    n2073 = property on="Figure_axis" class="Arr (strict)"("Value"=string[] [] ("Figure_axis_string")) -> ()  [unwired: 2 in, 2 out]
                  }
                  frame #1 {
                    w2617 = "Teslatron_iPS_OutputField" ("V_sweep")
                    n2074 = Build Array(w2617) -> (w2618:string[])
                    n2075 = Concatenate Strings(w2617, "\t") -> (w2620:string)
                    n2076 = property on="Figure_axis" class="Arr (strict)"("Value"=w2618) -> ()  [unwired: 2 in, 2 out]
                    n2077 = property on="data_caption" class="Str"("Value"=w2620) -> ()  [unwired: 2 in, 2 out]
                  }
                }
              }
              frame "iTC" {
                n2078 = stacked-sequence {
                  frame #0 {
                    n2079 = property on="data_caption" class="Str"("Value"="") -> ()  [unwired: 2 in, 2 out]
                    n2080 = property on="Figure_axis" class="Arr (strict)"("Value"=string[] ["", "SR830_1_ip", "SR830_1_oop", "SR830_2_ip", "SR830_2_oop", "2461_meas_v", "2461_meas_i", "2636A_smua_v", "2636A_smua_i", "formula"] ("Figure_axis")) -> ()  [unwired: 2 in, 2 out]
                  }
                  frame #1 {
                    w2625 = "Teslatron_iTC_Temp"
                    n2081 = Build Array(w2625) -> (w2624:string[])
                    n2082 = Concatenate Strings(w2625, "\t") -> (w2623:string)
                    n2083 = property on="data_caption" class="Str"("Value"=w2623) -> ()  [unwired: 2 in, 2 out]
                    n2084 = property on="Figure_axis" class="Arr (strict)"("Value"=w2624) -> ()  [unwired: 2 in, 2 out]
                  }
                }
              }
            }
            n2085 = case shown="True" w2574 {
              frame False {
              }
              frame True {
                # "opens session for 2636a system sourcemeter"
                n2086 = local read "2336A addr"() -> (w2627:refnum<visa-resource-name>)
                n2087 = VISA Open(VISA resource name=w2627) -> ()  [unwired: 4 in, 2 out]
              }
            }
          }
          frame #1 {
            # "0 = SR830_1_ip\n1 = SR830_1_oop\n2 = SR830_2_ip\n3 = SR830_2_oop\n4 = SR830_3_ip\n5 = SR830_3_oop\n6 = SR830_4_ip \n7 = SR830_4_oop \n8= 2400_1_v \n9 = 2400_1_i \n10 = 2400_2_v\n11 = 2400_2_i \n12 = 2400_3_v \n13 = 2400_3_i \n14 = 2182A_1_ch1 \n15 = 2182A_1_ch2 \n16 = 2182A_2_ch1 \n17 = 2182A_2_ch2\n18 = 2182A_3_ch1 \n19 = 2182A_3_ch2 \n20 = 2182A_4_ch1 \n21 = 2182A_4_ch2 \n22 = 2636A_smua_v \n23 = 2636A_smua_i \n24 = 2636A_smub_v \n25 = 2636A_smub_i \n26 = time\n27 = iPS_120\n28 = iTC _sample_T\n29 = iTC _CH_A\n30=iTC_CH_B\n31 = Step_Value"
            # "this part constructs the first (text) line for the data file with names of all measured variables,\nalso constructs a text array contaning names of all measured variable for the \"ring\" (so parameter can be selected and plotted)"
            n2088 = stacked-sequence {
              tunnel: [w2628 _ _ _ _ _ _ _ _ _ _ _ _ _ _ _ _ _ _ _ _ _ _ _ _ _ _ _ _ _ _] -> _
              frame #0 {
                # "SR830 1 in phase (SR830_1_ip)"
                n2089 = local read "SR830 1 ip"() -> (w2633:bool)
                n2090 = property on="Figure_axis" class="Arr (strict)"() -> ("Value"=w2630:string[])  [unwired: 2 in, 2 out]
                n2091 = property on="data_caption" class="Str"() -> ("Value"=w2632:string)  [unwired: 2 in, 2 out]
                n2092 = case shown="True" w2633 {
                  tunnel: w2632 -> [w2635 w2641]
                  tunnel: [w2635 w2640] -> w2631
                  tunnel: w2630 -> [w2634 w2638]
                  tunnel: [w2634 w2636] -> w2629
                  frame False {
                    # "not measure SR830 1 in phase signal (SR830_1_ip)"
                  }
                  frame True {
                    w2637 = "SR830_1_ip"
                    # "measure SR830 1 in phase signal (SR830_1_ip)"
                    n2093 = local read "SR830 1 addr"() -> (w2642:u8)
                    n2094 = Number To Decimal String(number=w2642) -> (decimal integer string=w2643:string)  [unwired: 1 in]
                    n2095 = GPIB Clear(3:w2643) -> ()  [unwired: 1 in, 2 out]
                    n2096 = Build Array (concatenate)(w2638, w2637) -> (w2636:string[])
                    n2097 = Concatenate Strings(w2641, w2637, "\t") -> (w2640:string)
                  }
                }
                n2098 = property on="Figure_axis" class="Arr (strict)"("Value"=w2629) -> ()  [unwired: 2 in, 2 out]
                n2099 = property on="data_caption" class="Str"("Value"=w2631) -> (error out=w2628:errorcluster)  [unwired: 2 in, 1 out]
              }
              frame #1 {
                # "SR830 1 out of phase (SR830_1_oop)"
                n2100 = local read "SR830 1 oop"() -> (w2648:bool)
                n2101 = property on="Figure_axis" class="Arr (strict)"() -> ("Value"=w2645:string[])  [unwired: 2 in, 2 out]
                n2102 = property on="data_caption" class="Str"() -> ("Value"=w2647:string)  [unwired: 2 in, 2 out]
                n2103 = case shown="False" w2648 {
                  tunnel: w2647 -> [w2650 w2656]
                  tunnel: [w2650 w2655] -> w2646
                  tunnel: w2645 -> [w2649 w2653]
                  tunnel: [w2649 w2651] -> w2644
                  frame False {
                    # "not measure SR830 1 out of phase signal (SR830_1_oop)"
                  }
                  frame True {
                    w2652 = "SR830_1_oop"
                    # "measure SR830 1 out of phase signal (SR830_1_oop)"
                    n2104 = local read "SR830 1 addr"() -> (w2657:u8)
                    n2105 = Number To Decimal String(number=w2657) -> (decimal integer string=w2658:string)  [unwired: 1 in]
                    n2106 = GPIB Clear(3:w2658) -> ()  [unwired: 1 in, 2 out]
                    n2107 = Build Array (concatenate)(w2653, w2652) -> (w2651:string[])
                    n2108 = Concatenate Strings(w2656, w2652, "\t") -> (w2655:string)
                  }
                }
                n2109 = property on="Figure_axis" class="Arr (strict)"("Value"=w2644) -> ()  [unwired: 2 in, 2 out]
                n2110 = property on="data_caption" class="Str"("Value"=w2646) -> ()  [unwired: 2 in, 2 out]
              }
              frame #2 {
                # "SR830 2 in phase (SR830_2_ip)"
                n2111 = local read "SR830 2 ip"() -> (w2663:bool)
                n2112 = property on="Figure_axis" class="Arr (strict)"() -> ("Value"=w2660:string[])  [unwired: 2 in, 2 out]
